vi "Configure Reporting.vi"(7 "Custom Reporting Plugin":string, 8 "error in (no error)":errorcluster, 10 "Path":path, 11 "Execution API In":refnum<class "Execution API.lvclass">) -> (0 "error out":errorcluster, 3 "Execution API Out":refnum<class "Execution API.lvclass">)   [LabVIEW 2020, in "Execution API.lvclass"]
doc: "Configure reporting path and toggle automatic report generation.\nIf you have a custom reporting plugin, it can be used by specifying the name of the report class. The report plugin must be installed as defined in LUnit documentation."
uses:
  Execution API.lvclass
  Plugins/Report/Report.lvclass
  C:/git/astemes-lunit/source/Framework/Plugin/Plugin.lvclass
  Execution API.lvclass/Execution API.ctl
  Plugin Loader/Plugin Loader.lvclass
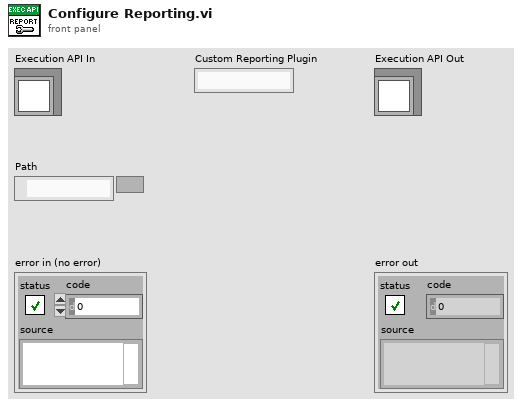
[diagram p1: front panel]
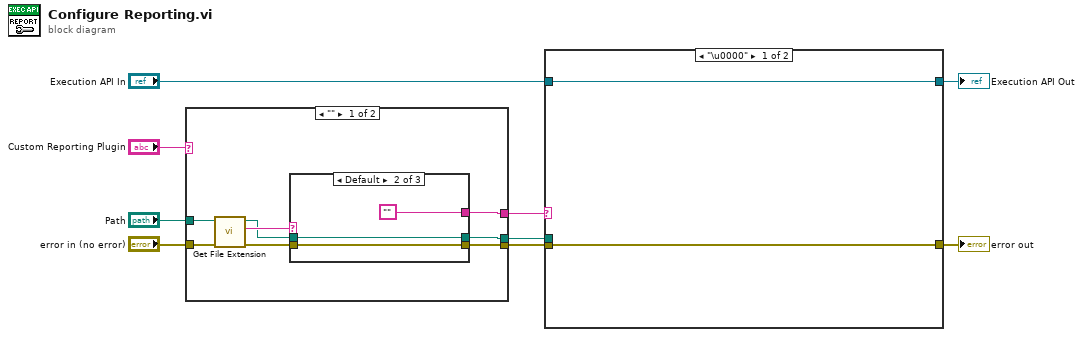
[diagram p0: block diagram]
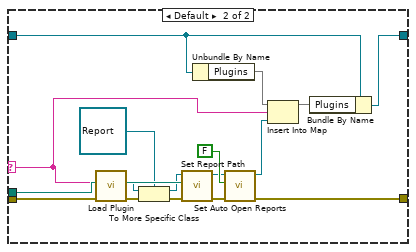
[diagram p2: hidden frame]
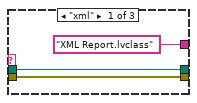
[diagram p3: hidden frame]
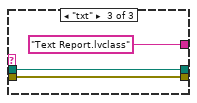
[diagram p4: hidden frame]
diagram:
  n1 = case shown="\"\"" "Custom Reporting Plugin" {
    selector: "Custom Reporting Plugin" -> [_ w27]
    tunnel: "Path" -> [w17 w28]
    tunnel: "error in (no error)" -> [w15 w29]
    tunnel: [w13 w29] -> w5
    tunnel: [w10 w28] -> w3
    tunnel: [w11 w27] -> w2
    frame "" {
      n2 = call <vilib>:"Get File Extension.vi"("error in (no error)"=w15, "file"=w17) -> ("error out"=w14:errorcluster, "lowercase file extension"=w16:string, "dup file"=w12:path)  [unwired: 5 in, 2 out]
      n3 = case shown="Default" w16 {
        tunnel: w14 -> [w20 w23 w26]
        tunnel: [w20 w23 w26] -> w13
        tunnel: w12 -> [w18 w21 w24]
        tunnel: ["XML Report.lvclass" ("Plugin") "" ("Plugin") "Text Report.lvclass" ("Plugin")] -> w11
        tunnel: [w18 w21 w24] -> w10
        frame "xml" {
        }
        frame Default {
        }
        frame "txt" {
        }
      }
    }
    frame Default {
    }
  }
  n4 = case shown="\"\"" w2 {
    selector: w2 -> [_ w44]
    tunnel: [w31 w48] -> w6
    tunnel: w5 -> [w30 w47]
    tunnel: [w30 w46] -> w4
    tunnel: w3 -> [_ w45]
    tunnel: "Execution API In" -> [w31 w32]
    frame "\u0000" {
    }
    frame Default {
      n5 = call "Load Plugin.vi"("error in (no error)"=w47, "Plugin"=w44) -> ("error out"=w38:errorcluster, "Plugin"=w35:refnum<class "Plugin.lvclass">)  [unwired: 8 in]
      n6 = To More Specific Class(target class=refnum<class "Report.lvclass"> refnum ("Report Out"), reference=w35, error in=w38) -> (specific class reference=w33:refnum<class "Report.lvclass">, error out=w36:errorcluster)
      n7 = call "Set Report Path.vi"("error in (no error)"=w36, "Report Path"=w45, "Report In"=w33) -> ("error out"=w37:errorcluster, "Report Out"=w41:refnum<class "Report.lvclass">)  [unwired: 7 in]
      n8 = Unbundle By Name(w32) -> ("Plugins"=w40:map{string, refnum<class "Plugin.lvclass">})
      n9 = call "Set Auto Open Reports.vi"("error in (no error)"=w37, "Open Generated Reports?"=FALSE, "Report In"=w41) -> ("error out"=w46:errorcluster, "Report Out"=w42:refnum<class "Report.lvclass">)  [unwired: 7 in]
      n10 = Insert Into Map(map in=w40, key=w44, value=w42) -> (map out=w39:map{string, refnum<class "Plugin.lvclass">})  [unwired: 2 out]
      n11 = Bundle By Name(cluster=w32, "Plugins"=w39) -> (w48:refnum<class "Execution API.lvclass">)
    }
  }
  "error out" <- w4
  "Execution API Out" <- w6
